vi "TCPConnectSendRead.vi"(2 "数据输入":string, 3 "读取的字节":i32=500, 4 "远程端口或服务名称":u16, 5 "地址":string) -> (0 "错误输出":errorcluster, 1 "数据输出":string)   [LabVIEW 2020]
panel:
  out "发送超时(ms)":i32=6000
  in  "读取超时(ms)":i32=6000
  in  "连接超时(ms)":i32=6000
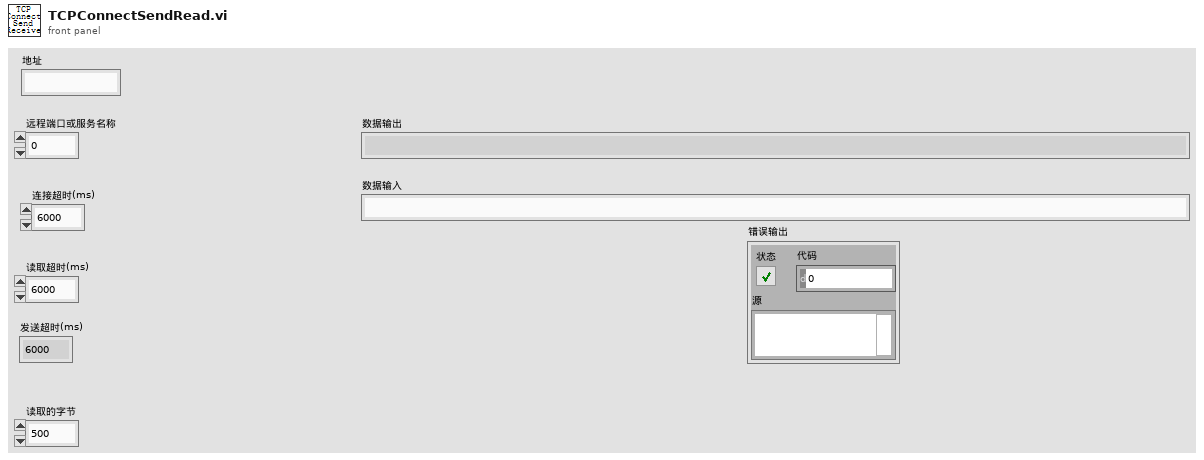
[diagram p1: front panel]
types:
  T1 = enum16{"Standard", "Buffered", "CRLF", "Immediate"}
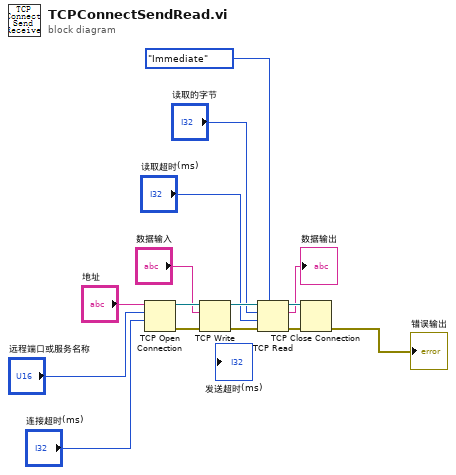
[diagram p0: block diagram]
diagram:
  n1 = TCP Open Connection(address="地址", remote port or service name="远程端口或服务名称", timeout ms (60000)="连接超时(ms)") -> (connection ID=w15:refnum<k5>, error out=w12:errorcluster)  [unwired: 2 in]
  n2 = TCP Write(connection ID=w15, data in="数据输入", error in (no error)=w12) -> (connection ID out=w14:refnum<k5>, error out=w11:errorcluster)  [unwired: 1 in, 1 out]
  n3 = TCP Read(connection ID=w14, bytes to read="读取的字节", error in (no error)=w11, 7:T1."Immediate" ("模式（标准）"), 9:"读取超时(ms)") -> (connection ID out=w13:refnum<k5>, data out=→"数据输出":string, error out=w10:errorcluster)
  n4 = TCP Close Connection(connection ID=w13, error in (no error)=w10) -> (error out=→"错误输出":errorcluster)  [unwired: 1 in, 1 out]
